vi "Seconds to Time.vi"(11 "Time Goal (s)":dbl=1.0 format="%#.6f") -> (0 "Seconds":dbl=1.0 format="%#.6f", 1 "Minutes":dbl=1.0, 2 "Hours":dbl=1.0, 3 "Days":dbl=1.0)   [LabVIEW 2021, in "Timer-API.lvlib" / "Timer Session.lvclass"]
doc: "Calculate days, hours, minutes and seconds from seconds."
uses:
  Timer Session.lvclass
  Timer Session.lvclass/Timer Session.ctl
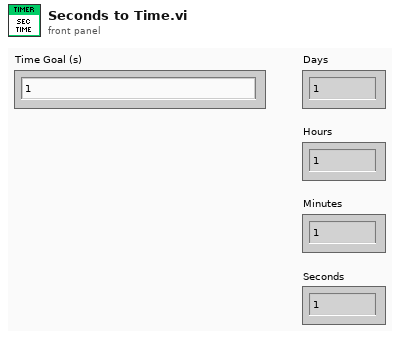
[diagram p1: front panel]
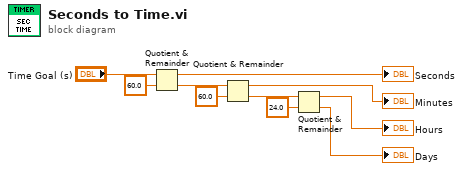
[diagram p0: block diagram]
diagram:
  n1 = Quotient & Remainder(x="Time Goal (s)", y=60.0) -> (x-y*floor(x/y)=→"Seconds":dbl, floor(x/y)=w7:dbl)
  n2 = Quotient & Remainder(x=w7, y=60.0) -> (x-y*floor(x/y)=→"Minutes":dbl, floor(x/y)=w3:dbl)
  n3 = Quotient & Remainder(x=w3, y=24.0) -> (x-y*floor(x/y)=→"Hours":dbl, floor(x/y)=→"Days":dbl)
